vi "make_axes_labels_number_generate.vi"(0 "from":dbl, 1 "Merged Array Out":T1(array[cluster]), 2 "Reverse?":bool, 5 "to":dbl, 7 "Font Size":dbl min=-1.7976931348623157e+308 max=1.7976931348623157e+308, 9 "width":dbl, 11 "height":dbl, 12 "Color Box":u32(colorbox)=4863, 13 "Right justified":bool, 14 "Draw Last Label?":bool=TRUE, 15 "Draw First Label?":bool=TRUE) -> (4 "Scene:New Object":refnum<vi>, 8 "Max Width":dbl)   [LabVIEW 2020, in "3DPC_SurfacePlot.xctl"]
uses:
  <vilib>/Native 3D Graph/xcontrol/3DPC_SurfacePlot.xctl
  <vilib>/picture/3D Picture Control/Object/Create Object (name).vi
  <vilib>/picture/3D Picture Control/NI_3D Picture Control.lvlib
panel:
  out "Draw First Label Copy":bool=TRUE
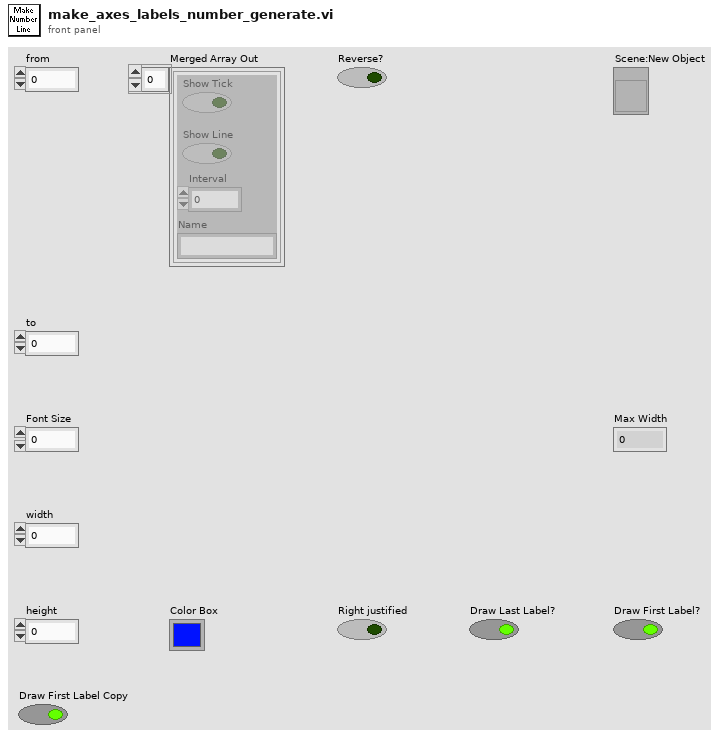
[diagram p1: front panel]
types:
  T1 = cluster{"Show Tick":bool, "Show Line":bool, "Interval":sgl, "Name":string}[]
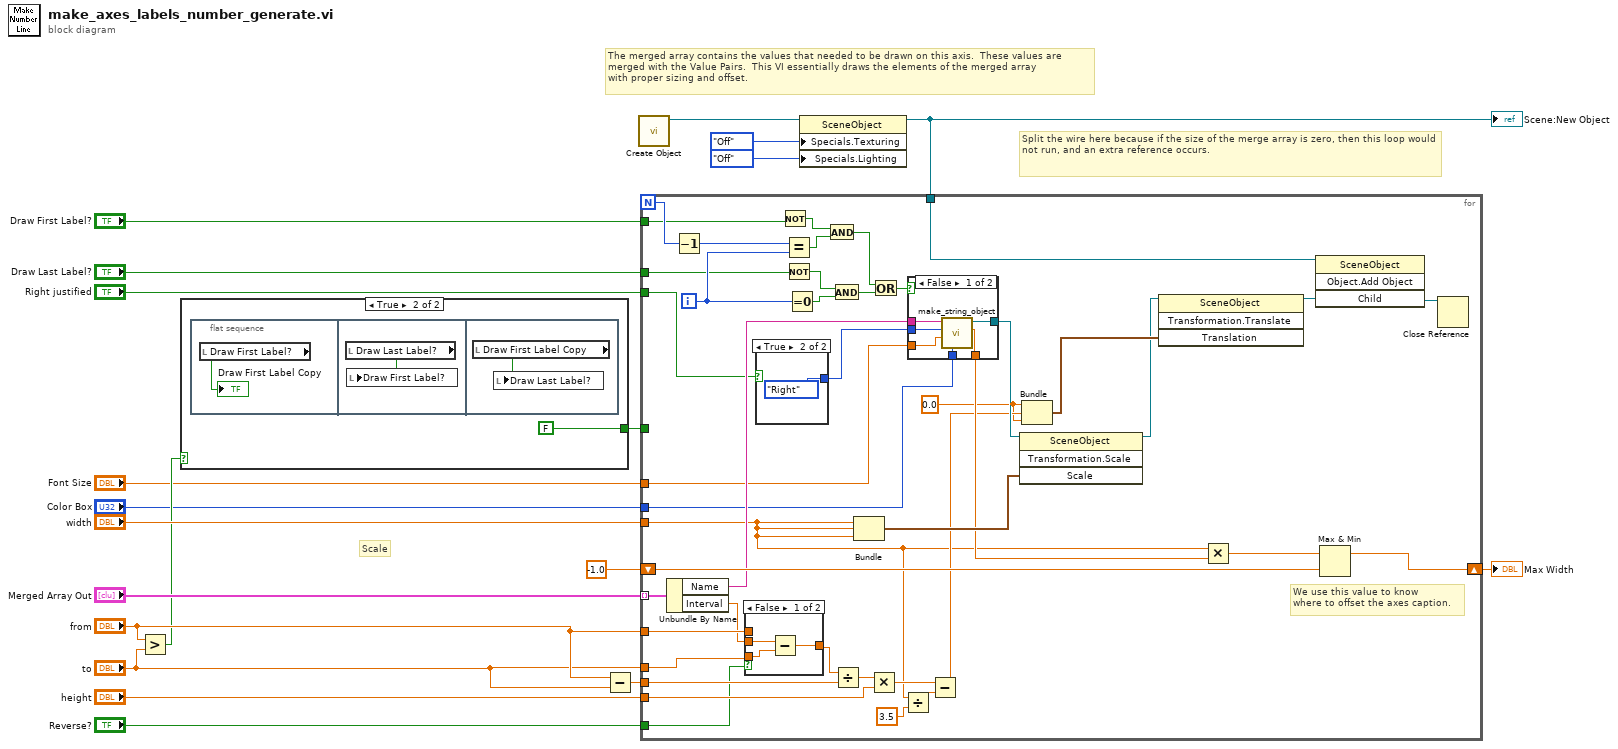
[diagram p0: block diagram]
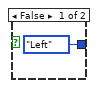
[diagram p2: hidden frame]
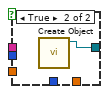
[diagram p3: hidden frame]
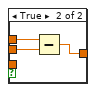
[diagram p4: hidden frame]
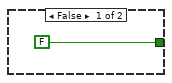
[diagram p5: hidden frame]
diagram:
  # "Split the wire here because if the size of the merge array is zero, then this loop would not run, and an extra reference occurs."
  # "The merged array contains the values that needed to be drawn on this axis.  These values are\nmerged with the Value Pairs.  This VI essentially draws the elements of the merged array\nwith proper sizing and offset."
  # "Scale"
  n1 = Greater?(x="from", y="to") -> (0:w7:bool)
  n2 = case shown="True" w7 {
    tunnel: [FALSE ("Right justified") FALSE ("Right justified")] -> w6
    frame False {
    }
    frame True {
      n3 = flat-sequence {
        frame #0 {
          n4 = local read "Draw First Label?"() -> (→"Draw First Label Copy":bool)
        }
        frame #1 {
          n5 = local read "Draw Last Label?"() -> (w24:bool)
          n6 = local write "Draw First Label?"(w24) -> ()
        }
        frame #2 {
          n7 = local read "Draw First Label Copy"() -> (w25:bool)
          n8 = local write "Draw Last Label?"(w25) -> ()
        }
      }
    }
  }
  n9 = Subtract(x="from", y="to") -> (x-y=w13:dbl)
  n10 = call-poly <vilib>:"Create Object.vi"() -> ("Scene:New Object"=w18:refnum<vi>)  [unwired: 10 in, 1 out]
  n11 = property class="SceneObject"(reference=w18, "Specials.Texturing"=enum16{"Inherit Value", "Off", "On"}."Off" ("Specials:Texturing"), "Specials.Lighting"=enum16{"Inherit Value", "Off", "On"}."Off" ("Specials:Lighting")) -> (reference out=w10:refnum<vi>)  [unwired: 1 in, 1 out]
  "Scene:New Object" <- w10
  n12 = for {
    N -> [w40]
    tunnel: w10 -> [w68]
    tunnel: "height" -> [w57]
    tunnel: "width" -> [w43]
    shift-right: [w61] -> w14
    shift-left: -1.0 -> [w62]
    tunnel: "Merged Array Out" -> [w55] mode=indexing
    tunnel: "from" -> [w51]
    tunnel: "to" -> [w49]
    tunnel: w13 -> [w58]
    tunnel: "Reverse?" -> [w48]
    tunnel: w6 -> [_]
    tunnel: "Draw First Label?" -> [w30]
    tunnel: "Draw Last Label?" -> [w29]
    tunnel: "Right justified" -> [w28]
    tunnel: "Color Box" -> [w27]
    tunnel: "Font Size" -> [w26]
    i -> [w39]
    w32 = sgl 0.0 ("Y")
    # "We use this value to know\nwhere to offset the axes caption."
    n13 = Unbundle By Name(w55) -> ("Name"=w54:string, "Interval"=w50:sgl)
    n14 = Decrement(x=w40) -> (x-1=w41:i32)
    n15 = case shown="False" w48 {
      tunnel: [w78 w83] -> w53
      tunnel: w51 -> [_ w82]
      tunnel: w50 -> [w80 w81]
      tunnel: w49 -> [w79 _]
      frame False {
        n16 = Subtract(x=w80, y=w79) -> (x-y=w78:dbl)
      }
      frame True {
        n17 = Subtract(x=w82, y=w81) -> (x-y=w83:dbl)
      }
    }
    n18 = case shown="True" w28 {
      tunnel: [enum8{"Left", "Right", "Center"}."Left" ("Alignment:Horizontal") enum8{"Left", "Right", "Center"}."Right" ("Alignment:Horizontal")] -> w31
      frame False {
      }
      frame True {
      }
    }
    n19 = Not(x=w30) -> (.not. x?=w38:bool)
    n20 = Equal?(x=w41, y=w39) -> (x = y?=w37:bool)
    n21 = Not(x=w29) -> (.not. x?=w46:bool)
    n22 = Equal To 0?(x=w39) -> (x = 0?=w47:bool)
    n23 = And(x=w38, y=w37) -> (x .and. y?=w36:bool)
    n24 = And(x=w46, y=w47) -> (x .and. y?=w35:bool)
    n25 = Divide(x=w53, y=w58) -> (x/y=w56:dbl)
    n26 = Bundle("width"=w43, "width"=w43, "width"=w43) -> (w66:cluster{"width":dbl, "width":dbl, "width":dbl})  [unwired: 1 out]
    n27 = Multiply(x=w56, y=w57) -> (x*y=w52:dbl)
    n28 = Or(x=w36, y=w35) -> (x .or. y?=w34:bool)
    n29 = Divide(x=w43, y=3.5) -> (x/y=w44:dbl)
    n30 = case shown="False" w34 {
      tunnel: w27 -> [w76 _]
      tunnel: [w75 w77] -> w65
      tunnel: [w74 _] -> w60
      tunnel: w54 -> [w73 _]
      tunnel: w26 -> [w72 _]
      tunnel: w31 -> [w71 _]
      frame False {
        n31 = call <vilib>:"make_string_object.vi"("Color"=w76, "Font Size"=w72, "Alignment:Horizontal"=w71, "String"=w73) -> ("Width"=w74:dbl, "String Object Out"=w75:refnum<vi>)  [unwired: 6 out]
      }
      frame True {
        n32 = call-poly <vilib>:"Create Object.vi"() -> ("Scene:New Object"=w77:refnum<vi>)  [unwired: 10 in, 1 out]
      }
    }
    n33 = Subtract(x=w52, y=w44) -> (x-y=w45:dbl)
    n34 = invoke class="SceneObject" method="Transformation.Scale"(reference=w65, "Scale"=w66) -> (reference out=w64:refnum<vi>)  [unwired: 2 in, 3 out]
    n35 = Bundle("Y"=w32, w45, "Y"=w32) -> (w67:cluster{"Y":sgl, dbl, "Y":sgl})  [unwired: 1 out]
    n36 = invoke class="SceneObject" method="Transformation.Translate"(reference=w64, "Translation"=w67) -> (reference out=w63:refnum<vi>)  [unwired: 2 in, 3 out]
    n37 = Multiply(x=w43, y=w60) -> (x*y=w59:dbl)
    n38 = invoke class="SceneObject" method="Object.Add Object"(reference=w68, "Child"=w63) -> ("Child"=w33:refnum<vi>)  [unwired: 2 in, 3 out]
    n39 = Max & Min(x=w59, y=w62) -> (max(x,y)=w61:dbl)  [unwired: 1 out]
    n40 = Close Reference(reference=w33) -> ()  [unwired: 1 in, 1 out]
  }
  "Max Width" <- w14
